vi "SAS_CmdStr.vi"(1 "SAS0E0":T1={"实际方向盘转向角"=-780.0, "方向盘转角速度"=0, "方向盘转向标定位"=FALSE, "SASFailureStatus"=FALSE, "计数"=0} {"方向盘转角速度" min=0 max=1016 step=4 scale=0.0..1016.0; "实际方向盘转向角" min=-780.0 max=779.9 step=0.03124 scale=-780.0..779.9 scale format="%6.1f"}) -> (0 "CmdStr":string)   [LabVIEW 2013]
uses:
  SAS_0E0.ctl
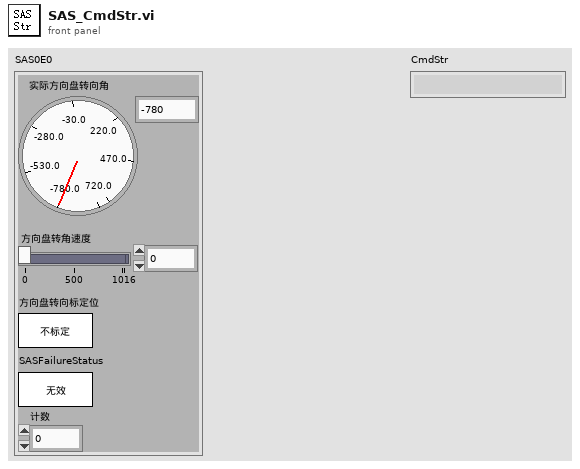
[diagram p1: front panel]
types:
  T1 = typedef "SAS_0E0.ctl" = cluster{"实际方向盘转向角":dbl, "方向盘转角速度":i32, "方向盘转向标定位":bool, "SASFailureStatus":bool, "计数":u8}
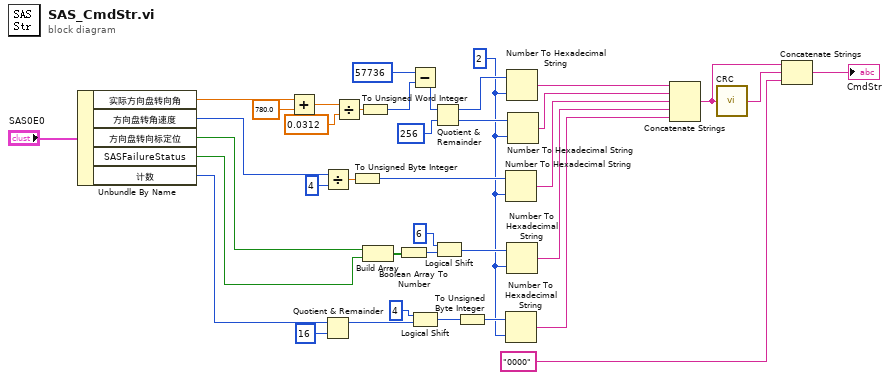
[diagram p0: block diagram]
diagram:
  w1 = 2
  n1 = Unbundle By Name("SAS0E0") -> ("实际方向盘转向角"=w6:dbl, "方向盘转角速度"=w5:i32, "方向盘转向标定位"=w4:bool, "SASFailureStatus"=w3:bool, "计数"=w2:u8)
  n2 = Add(x=w6, y=780.0) -> (x+y=w32:dbl)
  n3 = Divide(x=w5, y=4) -> (x/y=w37:dbl)
  n4 = Quotient & Remainder(x=w2, y=u8 16) -> (x-y*floor(x/y)=w11:u8)  [unwired: 1 out]
  n5 = Divide(x=w32, y=0.0312) -> (x/y=w30:dbl)
  n6 = To Unsigned Byte Integer(number=w37) -> (unsigned 8bit integer=w24:u8)
  n7 = To Unsigned Word Integer(number=w30) -> (unsigned 16bit integer=w17:u16)
  n8 = Build Array(w4, w3) -> (w36:bool[])
  n9 = Boolean Array To Number(Boolean array=w36) -> (number=w35:u32)
  n10 = Subtract(x=u16 57736, y=w17) -> (x-y=w16:u16)
  n11 = Logical Shift(y=u8 4, x=w11) -> (x << y=w14:u8)
  n12 = Quotient & Remainder(x=w16, y=u16 256) -> (x-y*floor(x/y)=w27:u16, floor(x/y)=w28:u16)
  n13 = Logical Shift(y=u8 6, x=w35) -> (x << y=w22:u32)
  n14 = To Unsigned Byte Integer(number=w14) -> (unsigned 8bit integer=w12:u8)
  n15 = Number To Hexadecimal String(1:w1, 2:w24) -> (0:w23:string)
  n16 = Number To Hexadecimal String(1:w1, 2:w12) -> (0:w15:string)
  n17 = Number To Hexadecimal String(1:w1, 2:w27) -> (0:w26:string)
  n18 = Number To Hexadecimal String(1:w1, 2:w22) -> (0:w21:string)
  n19 = Number To Hexadecimal String(1:w1, 2:w28) -> (0:w25:string)
  n20 = Concatenate Strings(w26, w25, w23, w21, w15) -> (w20:string)
  n21 = call "CRC.vi"("StrIn"=w20) -> ("StrOut"=w19:string)
  n22 = Concatenate Strings(w20, w19, "0000") -> (→"CmdStr":string)
